vi "arduinoInit.vi"(3 "error in (no error)":errorcluster, 4 "arduinoSerial in":T2 {"Serial Settings 2"."flow control" items=["None"=0, "XON/XOFF"=1, "RTS/CTS"=2, "DTR/DSR"=4]; "Serial Settings 2"."stop bits" items=["1.0"=10, "1.5"=15, "2.0"=20]; "Serial Settings 2"."data bits" min=5 max=8 step=1; "Serial Settings 2"."baud rate" items=["75"=75, "110"=110, "134"=134, "150"=150, "300"=300, "600"=600, "1200"=1200, "1800"=1800, "2400"=2400, "4800"=4800, "7200"=7200, "9600"=9600, "14400"=14400, "19200"=19200, "28800"=28800, "38400"=38400, "56000"=56000, "57600"=57600, "115200"=115200, "128000"=128000, "230400"=230400]}) -> (0 "error out":errorcluster, 1 "arduinoSerial out":T2 {"Serial Settings 2"."flow control" items=["None"=0, "XON/XOFF"=1, "RTS/CTS"=2, "DTR/DSR"=4]; "Serial Settings 2"."stop bits" items=["1.0"=10, "1.5"=15, "2.0"=20]; "Serial Settings 2"."data bits" min=5 max=8 step=1; "Serial Settings 2"."baud rate" items=["75"=75, "110"=110, "134"=134, "150"=150, "300"=300, "600"=600, "1200"=1200, "1800"=1800, "2400"=2400, "4800"=4800, "7200"=7200, "9600"=9600, "14400"=14400, "19200"=19200, "28800"=28800, "38400"=38400, "56000"=56000, "57600"=57600, "115200"=115200, "128000"=128000, "230400"=230400]}, 2 "VISA resource name out":refnum<visa-resource-name>)   [LabVIEW 2021]
uses:
  Program Files/National Instruments/LabVIEW 2021/examples/Instrument IO/Serial/support/Serial - Settings.ctl
  <vilib>/Instr/_visa.llb/VISA Configure Serial Port (Instr).vi
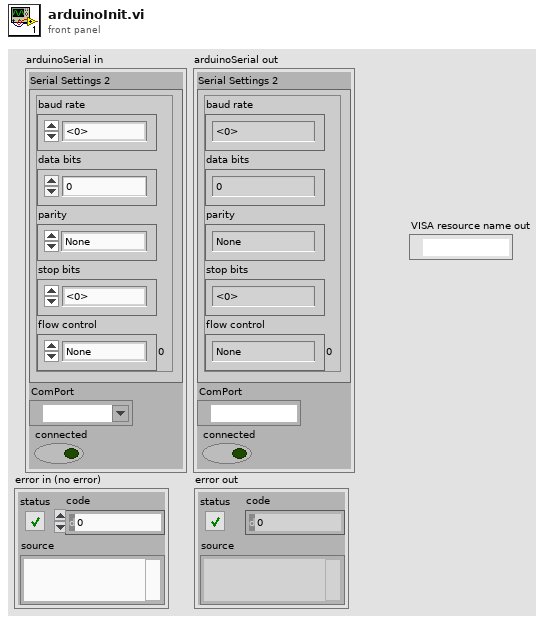
[diagram p1: front panel]
types:
  T1 = typedef "Serial - Settings.ctl" = cluster{"baud rate":u32, "data bits":u16, "parity":enum16{"None", "Odd", "Even", "Mark", "Space"}, "stop bits":u16, "flow control":u16}
  T2 = cluster{"Serial Settings 2":T1, "ComPort":refnum<visa-resource-name>, "connected":bool}
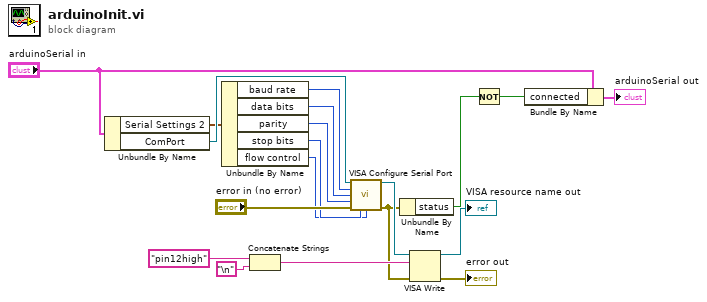
[diagram p0: block diagram]
diagram:
  n1 = Unbundle By Name("arduinoSerial in") -> ("Serial Settings 2"=w13:T1, "ComPort"=w14:refnum<visa-resource-name>)
  n2 = Unbundle By Name(w13) -> ("baud rate"=w12:u32, "data bits"=w11:u16, "parity"=w10:enum16{"None", "Odd", "Even", "Mark", "Space"}, "stop bits"=w9:u16, "flow control"=w8:u16)
  n3 = Concatenate Strings("pin12high", "\n") -> (w4:string)
  n4 = call-poly "VISA Configure Serial Port"("VISA resource name"=w14, "baud rate (9600)"=w12, "data bits (8)"=w11, "parity (0:none)"=w10, "error in (no error)"="error in (no error)", "stop bits (10: 1 bit)"=w9, "flow control (0:none)"=w8) -> ("VISA resource name out"=w7:refnum<visa-resource-name>, "error out"=w3:errorcluster)  [unwired: 2 in, 5 out]
  n5 = Unbundle By Name(w3) -> ("status"=w16:bool)
  n6 = VISA Write(VISA resource name=w7, write buffer=w4, error in (no error)=w3) -> (VISA resource name out=→"VISA resource name out":refnum<visa-resource-name>, error out=→"error out":errorcluster)  [unwired: 1 out]
  n7 = Not(x=w16) -> (.not. x?=w18:bool)
  n8 = Bundle By Name(cluster="arduinoSerial in", "connected"=w18) -> (→"arduinoSerial out":T2)
